vi "Console Send Message.vi"(0 "Message":string, 11 "error in (no error)":errorcluster) -> (15 "error out":errorcluster)   [LabVIEW 2026, in "MrcLib.lvlib"]
doc: "Appends the string message to the console and DS log."
uses:
  MrcLib.lvlib
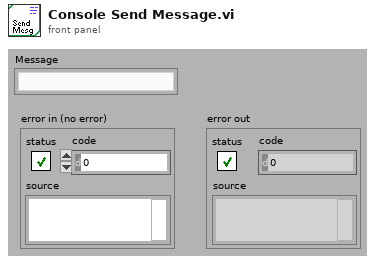
[diagram p1: front panel]
types:
  T1 = typedef "MRC String.ctl" = cluster{"pointer":u64, "length":u64}
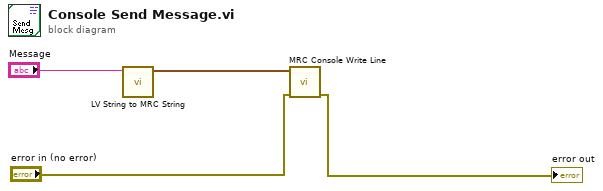
[diagram p0: block diagram]
diagram:
  n1 = call "LV String to MRC String.vi"("LV String"="Message") -> ("MRC String"=w3:T1)  [unwired: 10 in]
  n2 = call "MRC Console Write Line.vi"("error in (no error)"="error in (no error)", "line"=w3) -> ("error out"=→"error out":errorcluster)  [unwired: 9 in]
